vi "KolejkaMycia.vi"(8 "error in (no error)":errorcluster, 11 "Wash Options":T1) -> (0 "error out":errorcluster, 3 "Option Array":string[](array[string]))   [LabVIEW 2020]
uses:
  controls/WashOptions.ctl
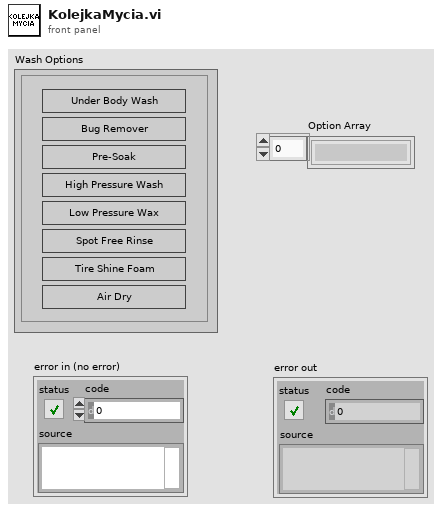
[diagram p1: front panel]
types:
  T1 = typedef "WashOptions.ctl" = cluster{"Bug Remover":bool, "Low Pressure Wax":bool, "High Pressure Wash":bool, "Pre-Soak":bool, "Spot Free Rinse":bool, "Air Dry":bool, "Under Body Wash":bool, "Tire Shine Foam":bool}
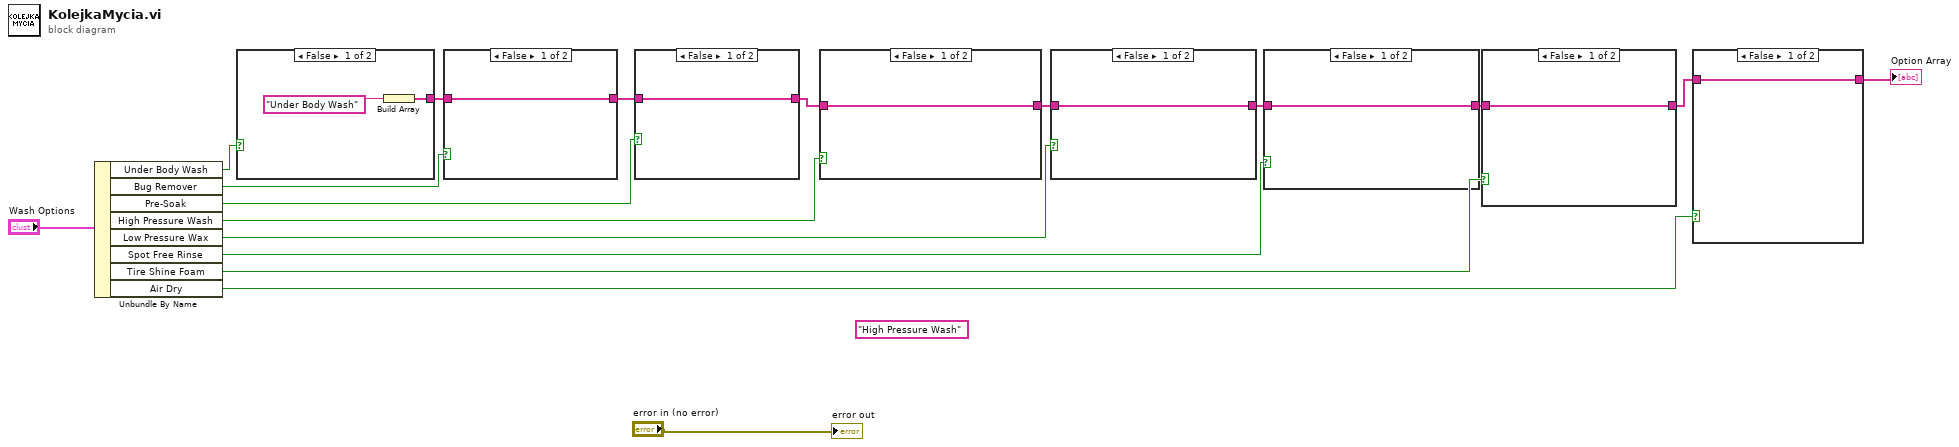
[diagram p0: block diagram]
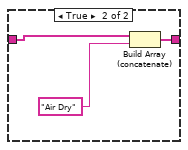
[diagram p2: hidden frame]
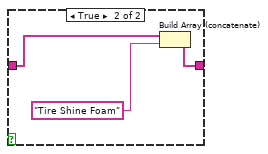
[diagram p3: hidden frame]
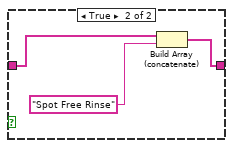
[diagram p4: hidden frame]
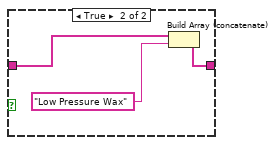
[diagram p5: hidden frame]
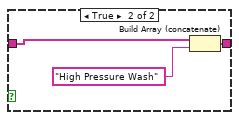
[diagram p6: hidden frame]
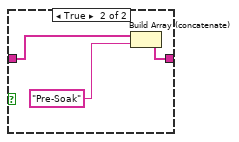
[diagram p7: hidden frame]
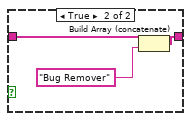
[diagram p8: hidden frame]
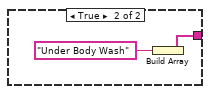
[diagram p9: hidden frame]
diagram:
  (unwired) "High Pressure Wash"
  n1 = Unbundle By Name("Wash Options") -> ("Under Body Wash"=w11:bool, "Bug Remover"=w17:bool, "Pre-Soak"=w18:bool, "High Pressure Wash"=w16:bool, "Low Pressure Wax"=w15:bool, "Spot Free Rinse"=w14:bool, "Tire Shine Foam"=w13:bool, "Air Dry"=w12:bool)
  n2 = case shown="False" w11 {
    tunnel: [w19 w21] -> w6
    frame False {
      n3 = Build Array("Under Body Wash") -> (w19:string[])
    }
    frame True {
      n4 = Build Array("Under Body Wash") -> (w21:string[])
    }
  }
  n5 = case shown="False" w17 {
    tunnel: w6 -> [w23 w26]
    tunnel: [w23 w25] -> w5
    frame False {
    }
    frame True {
      n6 = Build Array (concatenate)(w26, "Bug Remover") -> (w25:string[])
    }
  }
  n7 = case shown="False" w18 {
    tunnel: w5 -> [w27 w29]
    tunnel: [w27 w28] -> w4
    frame False {
    }
    frame True {
      n8 = Build Array (concatenate)(w29, "Pre-Soak") -> (w28:string[])
    }
  }
  n9 = case shown="False" w16 {
    tunnel: [w31 w33] -> w10
    tunnel: w4 -> [w31 w32]
    frame False {
    }
    frame True {
      n10 = Build Array (concatenate)(w32, "High Pressure Wash") -> (w33:string[])
    }
  }
  n11 = case shown="False" w15 {
    tunnel: w10 -> [w35 w38]
    tunnel: [w35 w36] -> w3
    frame False {
    }
    frame True {
      n12 = Build Array (concatenate)(w38, "Low Pressure Wax") -> (w36:string[])
    }
  }
  n13 = case shown="False" w14 {
    tunnel: w3 -> [w39 w41]
    tunnel: [w39 w40] -> w2
    frame False {
    }
    frame True {
      n14 = Build Array (concatenate)(w41, "Spot Free Rinse") -> (w40:string[])
    }
  }
  n15 = case shown="False" w13 {
    tunnel: w2 -> [w43 w45]
    tunnel: [w43 w44] -> w1
    frame False {
    }
    frame True {
      n16 = Build Array (concatenate)(w45, "Tire Shine Foam") -> (w44:string[])
    }
  }
  n17 = case shown="False" w12 {
    tunnel: [w47 w49] -> w8
    tunnel: w1 -> [w47 w48]
    frame False {
    }
    frame True {
      n18 = Build Array (concatenate)(w48, "Air Dry") -> (w49:string[])
    }
  }
  "Option Array" <- w8
  "error out" <- "error in (no error)"
